vi "Page_Info_Initialize.vi"(8 "error in (no error)":errorcluster, 9 "ctlReferences":T1, 11 "AB_Deploy_EXE in":refnum<class "AB_Deploy_EXE.lvclass">) -> (0 "error out":errorcluster, 3 "AB_Deploy_EXE out":refnum<class "AB_Deploy_EXE.lvclass">)   [LabVIEW 2020, in "AB_Deploy_EXE.lvclass"]
uses:
  <vilib>/AppBuilder/AB_Classes/DeployableEXE/AB_Deploy_EXE.lvclass
  <resource>/Framework/Providers/Builds/AppBuilder/AB_UI_Page_Info_References.ctl
  <resource>/Framework/Providers/Common/provcom_StringGlobals.vi
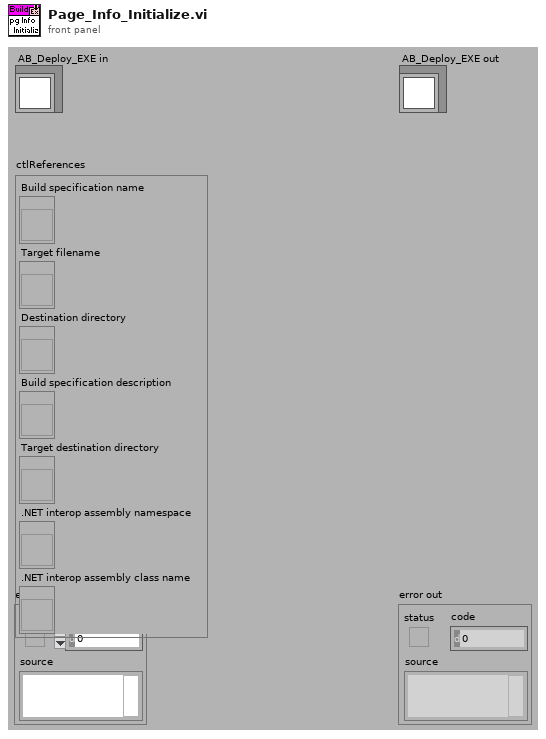
[diagram p1: front panel]
types:
  T1 = typedef "AB_UI_Page_Info_References.ctl" = cluster{"Build specification name":refnum<vi>, "Target filename":refnum<vi>, "Destination directory":refnum<vi>, "Build specification description":refnum<vi>, "Target destination directory":refnum<vi>, ".NET interop assembly namespace":refnum<vi>, ".NET interop assembly class name":refnum<vi>}
  T2 = typedef "LVRectTypeDef.ctl" = cluster{"Left":i16, "Top":i16, "Right":i16, "Bottom":i16}
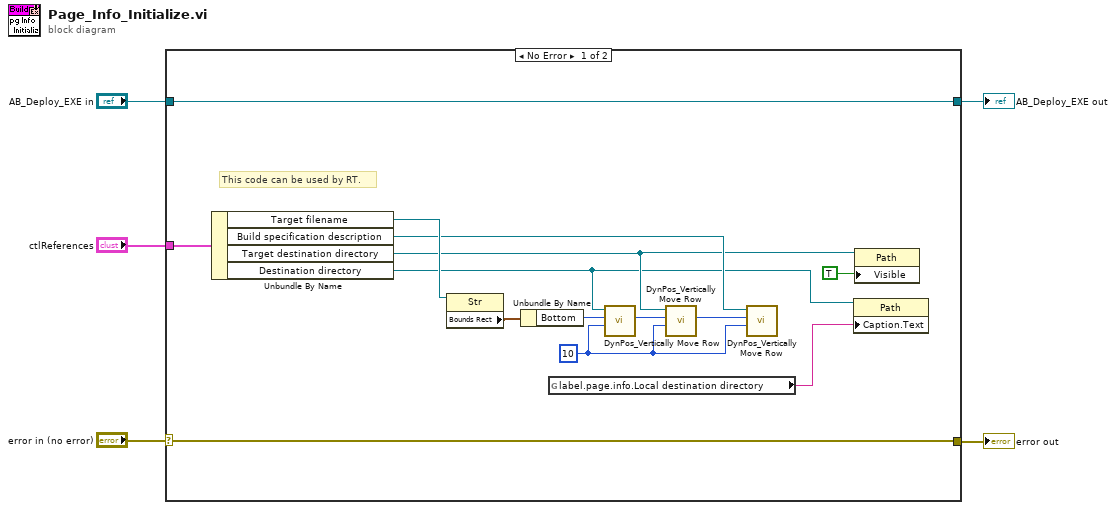
[diagram p0: block diagram]
diagram:
  n1 = case shown="No Error" "error in (no error)" {
    selector: "error in (no error)" -> [w8 w21]
    tunnel: [w8 w21] -> w4
    tunnel: "ctlReferences" -> [w19 _]
    tunnel: [w9 w20] -> w2
    tunnel: "AB_Deploy_EXE in" -> [w9 w20]
    frame No Error {
      w17 = 10 ("Pixel separation (6)")
      # "This code can be used by RT."
      n2 = Unbundle By Name(w19) -> ("Target filename"=w18:refnum<vi>, "Build specification description"=w12:refnum<vi>, "Target destination directory"=w10:refnum<vi>, "Destination directory"=w7:refnum<vi>)
      n3 = property class="Str"(reference=w18) -> ("Bounds Rect"=w13:T2)  [unwired: 1 in, 2 out]
      n4 = Unbundle By Name(w13) -> ("Bottom"=w14:i16)
      n5 = global read "provcom_StringGlobals.vi" "label.page.info.Local destination directory"() -> (w6:string)
      n6 = call <vilib>:"DynPos_Vertically Move Row.vi"("Pixel separation (6)"=w17, "Bottom of last control"=w14, "Control"=w7) -> ("Bottom pixel"=w15:i32)  [unwired: 7 in, 1 out]
      n7 = call <vilib>:"DynPos_Vertically Move Row.vi"("Pixel separation (6)"=w17, "Bottom of last control"=w15, "Control"=w10) -> ("Bottom pixel"=w16:i32)  [unwired: 7 in, 1 out]
      n8 = call <vilib>:"DynPos_Vertically Move Row.vi"("Pixel separation (6)"=w17, "Bottom of last control"=w16, "Control"=w12) -> ()  [unwired: 7 in, 2 out]
      n9 = property class="Path"(reference=w7, "Caption.Text"=w6) -> ()  [unwired: 1 in, 2 out]
      n10 = property class="Path"(reference=w10, "Visible"=TRUE) -> ()  [unwired: 1 in, 2 out]
    }
    frame Error {
    }
  }
  "error out" <- w4
  "AB_Deploy_EXE out" <- w2
